vi "terminate.vi"(8 "error in (no error)":errorcluster, 11 "YK090623DAQmxAnalogDetector in":refnum<class "DetectorYK090623DAQmxAnalog.lvclass">) -> (0 "error out":errorcluster, 3 "YK090623DAQmxAnalogDetector out":refnum<class "DetectorYK090623DAQmxAnalog.lvclass">)   [LabVIEW 2010, in "DetectorYK090623DAQmxAnalog.lvclass"]
doc: "The dynamic dispatch version of this VI terminates the plug-in object by releasing all of its resources."
uses:
  DetectorYK090623DAQmxAnalog.lvclass
  DetectorYK090623DAQmxAnalog.lvclass/DetectorYK090623DAQmxAnalog.ctl
  AnalogOut/AnalogOutDL101207DAQmx/AnalogOutDL101207DAQmx/AnalogOutDL101207DAQmx.lvclass
  GenericDetector/GenericDetector/GenericDetector.lvclass
  common/classes/ErrorController/ErrorController/class_data.vi
  common/classes/ErrorController/ErrorController/ErrorController.lvclass
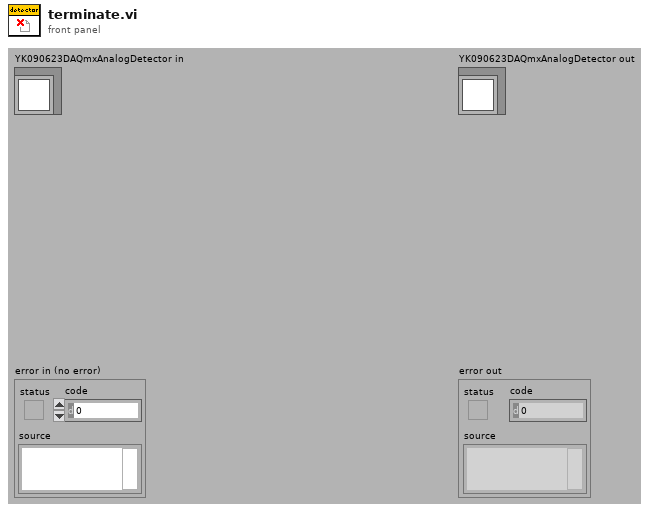
[diagram p1: front panel]
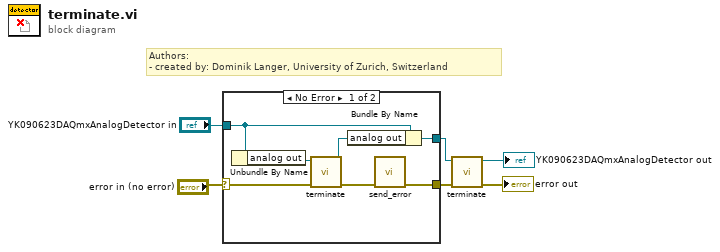
[diagram p0: block diagram]
diagram:
  # "Authors: \n- created by: Dominik Langer, University of Zurich, Switzerland"
  n1 = case shown="No Error" "error in (no error)" {
    selector: "error in (no error)" -> [w12 w14]
    tunnel: [w7 w14] -> w3
    tunnel: "YK090623DAQmxAnalogDetector in" -> [w10 w15]
    tunnel: [w9 w15] -> w1
    frame No Error {
      n2 = Unbundle By Name(w10) -> ("analog out"=w13:refnum<class "AnalogOutDL101207DAQmx.lvclass">)
      n3 = call-dynamic "terminate.vi"("error in (no error)"=w12, "DAQmxAnalogOut in"=w13) -> ("error out"=w8:errorcluster, "DAQmxAnalogOut out"=w11:refnum<class "AnalogOutDL101207DAQmx.lvclass">)  [unwired: 8 out]
      n4 = Bundle By Name(cluster=w10, "analog out"=w11) -> (w9:refnum<class "DetectorYK090623DAQmxAnalog.lvclass">)
      n5 = call "send_error.vi"("error in (no error)"=w8) -> ("error out"=w7:errorcluster)  [unwired: 10 in]
    }
    frame Error {
    }
  }
  n6 = call-parent "terminate.vi"("error in (no error)"=w3, "GenericPlugin in"=w1) -> ("error out"=→"error out":errorcluster, "GenericPlugin out"=→"YK090623DAQmxAnalogDetector out":refnum<class "DetectorYK090623DAQmxAnalog.lvclass">)  [unwired: 8 out]
